vi "Util Convert From Base64 and Store.vi"(8 "error in (no error)":errorcluster, 9 "file path":path, 10 "Write to File":bool, 11 "Base64 String":string) -> (0 "error out":errorcluster, 3 "String":string)   [LabVIEW 2010, in "chaosui-crest.lvlib"]
doc: "This VI converts a Base 64 string to its string equivalent. Base64 strings are commonly used in Internet protocols such as HTTP, SMTP, etc."
uses:
  chaosui-crest.lvlib
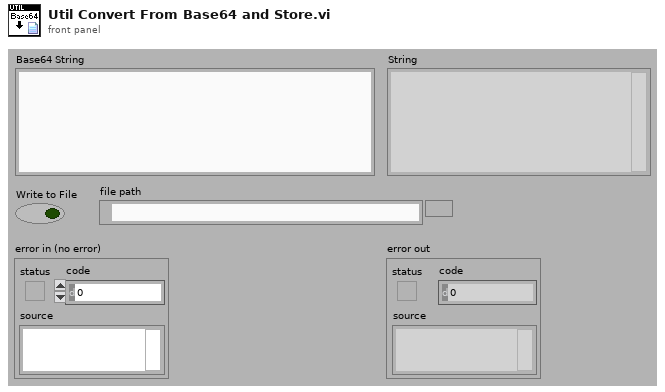
[diagram p1: front panel]
types:
  T1 = enum16{"open", "replace", "create", "open or create", "replace or create", "replace or create with confirmation"}
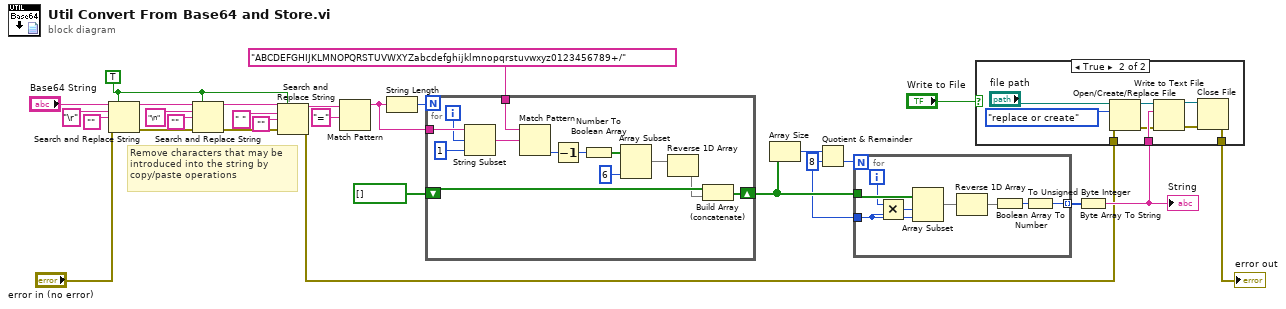
[diagram p0: block diagram]
diagram:
  w1 = TRUE ("replace all? (F)")
  w20 = 8 ("y")
  # "Remove characters that may be\nintroduced into the string by\ncopy/paste operations"
  n1 = Search and Replace String(replace all?=w1, input string="Base64 String", search string="\r" ("replace string (\"\")"), replace string="", error in="error in (no error)") -> (result string=w12:string, error out=w4:errorcluster)  [unwired: 5 out]
  n2 = Search and Replace String(replace all?=w1, input string=w12, search string="\n" ("replace string (\"\")"), replace string="", error in=w4) -> (result string=w6:string, error out=w7:errorcluster)  [unwired: 5 out]
  n3 = Search and Replace String(replace all?=w1, input string=w6, search string=" " ("replace string (\"\")"), replace string="", error in=w7) -> (result string=w5:string, error out=w2:errorcluster)  [unwired: 5 out]
  n4 = Match Pattern(string=w5, regular expression="=") -> (before substring=w25:string)  [unwired: 4 out]
  n5 = String Length(string=w25) -> (length=w28:i32)
  n6 = for {
    N: w28 -> [_]
    tunnel: w25 -> [w41]
    tunnel: "ABCDEFGHIJKLMNOPQRSTUVWXYZabcdefghijklmnopqrstuvwxyz0123456789+/" -> [w38]
    shift-right: [w31] -> w21
    shift-left: bool[] [] -> [w30]
    i -> [w39]
    n7 = String Subset(string=w41, offset (0)=w39, length (rest)=1 ("length (rest)")) -> (substring=w37:string)
    n8 = Match Pattern(string=w38, regular expression=w37) -> (offset past match=w36:i32)  [unwired: 4 out]
    n9 = Decrement(x=w36) -> (x-1=w35:i32)
    n10 = Number To Boolean Array(number=w35) -> (Boolean array=w34:bool[])
    n11 = Array Subset(array=w34, length=6) -> (w32:bool[])  [unwired: 1 in]
    n12 = Reverse 1D Array(array=w32) -> (reversed array=w29:bool[])
    n13 = Build Array (concatenate)(w30, w29) -> (w31:bool[])
  }
  n14 = Array Size(array=w21) -> (size(s)=w23:i32)
  n15 = Quotient & Remainder(x=w23, y=w20) -> (floor(x/y)=w22:i32)  [unwired: 1 out]
  n16 = for {
    N: w22 -> [_]
    tunnel: w21 -> [w49]
    tunnel: w20 -> [w48]
    tunnel: [w44] -> w19 mode=indexing
    i -> [w47]
    n17 = Multiply(x=w47, y=w48) -> (x*y=w42:i32)
    n18 = Array Subset(array=w49, index=w42, length=w48) -> (w46:bool[])
    n19 = Reverse 1D Array(array=w46) -> (reversed array=w43:bool[])
    n20 = Boolean Array To Number(Boolean array=w43) -> (number=w45:u32)
    n21 = To Unsigned Byte Integer(number=w45) -> (unsigned 8bit integer=w44:u8)
  }
  n22 = Byte Array To String(unsigned byte array=w19) -> (string=w17:string)
  "String" <- w17
  n23 = case shown="True" "Write to File" {
    tunnel: w17 -> [_ w59]
    tunnel: w2 -> [w50 w58]
    tunnel: [w50 w54] -> w10
    frame False {
    }
    frame True {
      n24 = Open/Create/Replace File(file path (use dialog)="file path", error in=w58, operation (0:open)=T1."replace or create") -> (refnum out=w53:refnum<file>, error out=w57:errorcluster)  [unwired: 4 out]
      n25 = Write to Text File(file (use dialog)=w53, text=w59, error in=w57) -> (refnum out=w55:refnum<file>, error out=w56:errorcluster)  [unwired: 1 in, 1 out]
      n26 = Close File(refnum=w55, error in=w56) -> (error out=w54:errorcluster)  [unwired: 1 out]
    }
  }
  "error out" <- w10
